vi "Gen - Init to Default.vi"(8 "Error in":errorcluster, 11 "This VI":refnum<vi>) -> (0 "Error out":errorcluster, 3 "This VI Copy":refnum<vi>)   [LabVIEW 2020]
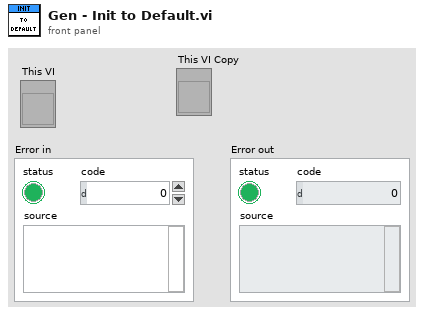
[diagram p1: front panel]
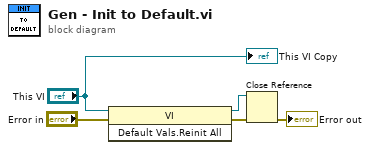
[diagram p0: block diagram]
diagram:
  n1 = invoke class="VI" method="Default Vals.Reinit All"(reference="This VI", error in="Error in") -> (reference out=w4:refnum<vi>, error out=w5:errorcluster)  [unwired: 1 in, 1 out]
  n2 = Close Reference(reference=w4, error in (no error)=w5) -> (error out=→"Error out":errorcluster)
  "This VI Copy" <- "This VI"
